vi "Get Error Message.vi"(8 "Error In":errorcluster, 10 "Actuator Type":string, 11 "Error Code":i32) -> (0 "Error Out":errorcluster, 3 "Error Message":string)   [LabVIEW 2023]
uses:
  <vilib>/Utility/file.llb/Read Delimited Spreadsheet (string).vi
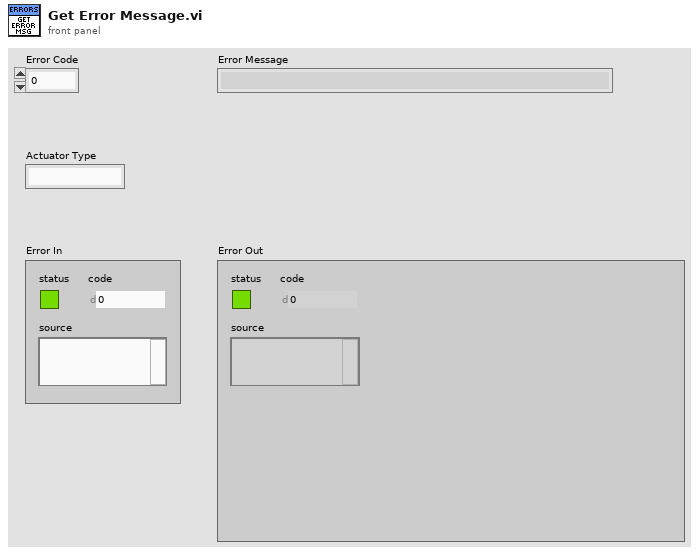
[diagram p1: front panel]
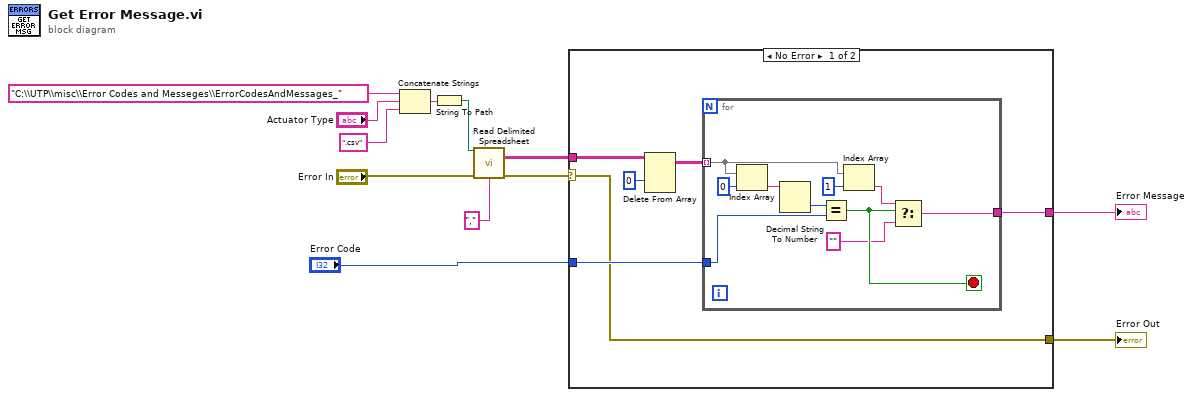
[diagram p0: block diagram]
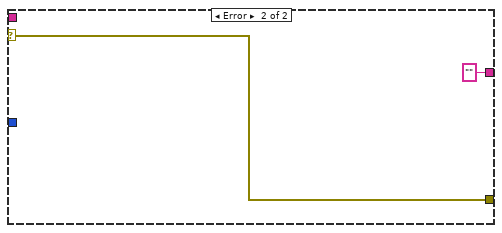
[diagram p2: hidden frame]
diagram:
  n1 = Concatenate Strings("C:\\UTP\\misc\\Error Codes and Messeges\\ErrorCodesAndMessages_", "Actuator Type", ".csv") -> (w2:string)
  n2 = String To Path(string=w2) -> (path=w1:path)
  n3 = call-poly <vilib>:"Read Delimited Spreadsheet.vi"("file path (dialog if empty)"=w1, "error in (no error)"="Error In", "delimiter (\\t)"="," ("delimiter (\\t)")) -> ("all rows"=w9:string[][], "error out"=w8:errorcluster)  [unwired: 7 in, 4 out]
  n4 = case shown="No Error" w8 {
    selector: w8 -> [w13 w29]
    tunnel: "Error Code" -> [w18 _]
    tunnel: w9 -> [w17 _]
    tunnel: [w14 "" ("f")] -> w7
    tunnel: [w13 w29] -> w6
    frame No Error {
      n5 = Delete From Array(array=w17, index (row)=0) -> (array with subset deleted=w15:string[][])  [unwired: 2 in, 1 out]
      n6 = for {
        tunnel: w15 -> [w24] mode=indexing
        tunnel: w18 -> [w25]
        tunnel: [w21] -> w14
        stop <- w20 stop-if-true
        n7 = Index Array(array=w24, index=0) -> (element=w27:string)
        n8 = Decimal String To Number(string=w27) -> (number=w26:i32)  [unwired: 2 in, 1 out]
        n9 = Equal?(x=w26, y=w25) -> (x = y?=w20:bool)
        n10 = Index Array(array=w24, index=1) -> (element=w22:string)
        n11 = Select(t=w22, s=w20, f="") -> (s? t:f=w21:string)
      }
    }
    frame Error {
    }
  }
  "Error Out" <- w6
  "Error Message" <- w7
